vi "Write and Read Multiple Registers.vi"(4 "read count":u16, 6 "read starting address":u16, 8 "error in":errorcluster, 9 "write values":u16[](array[numeric]), 10 "write starting address":u16, 11 "device data model in":refnum<class "Standard Data Model.lvclass">) -> (0 "error out":errorcluster, 1 "read values":u16[](array[numeric]), 3 "device data model out":refnum<class "Standard Data Model.lvclass">)   [LabVIEW 2013, in "Modbus Library - Advance.lvlib" / "Standard Data Model.lvclass"]
doc: "Writes and reads the values of multiple register values in series. The <b>write values</b> are inserted starting at <b>write starting address</b> and the returned <b>read values</b> consists of <b>read count</b> holding registers starting at <b>read starting address</b>."
uses:
  Standard Data Model.lvclass
  Standard Data Model.lvclass/Standard Data Model.ctl
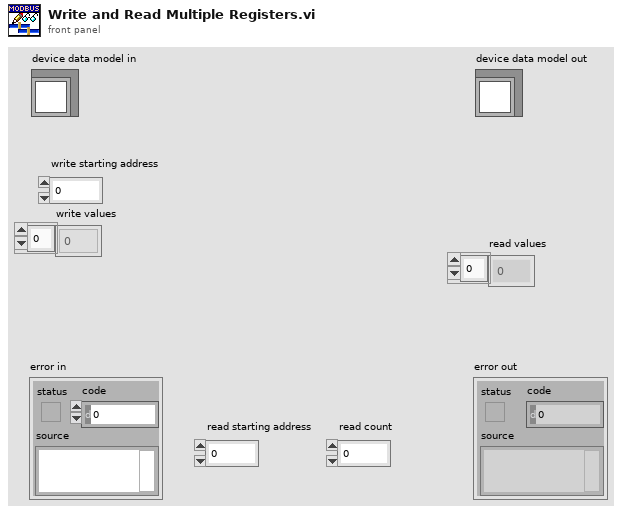
[diagram p1: front panel]
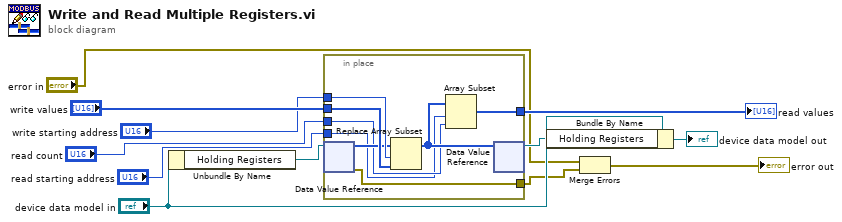
[diagram p0: block diagram]
diagram:
  n1 = Unbundle By Name("device data model in") -> ("Holding Registers"=w10:refnum<data-value>)
  n2 = in-place {
    in-place-border: "write values" -> [w20]
    in-place-border: "write starting address" -> [w19]
    in-place-border: [w16] -> w7
    in-place-border: "read count" -> [w15]
    in-place-border: "read starting address" -> [w14]
    in-place-border: [w13] -> w1
    n3 = in-place-dvr #1(w10) -> (w18:u16[], w13:errorcluster)
    n4 = Replace Array Subset(array=w18, new element=w20, index=w19) -> (w17:u16[])
    n5 = Array Subset(array=w17, index=w14, length=w15) -> (w16:u16[])
    n6 = in-place-dvr #1(w17) -> (w3:refnum<data-value>)  [unwired: 1 out]
  }
  "read values" <- w7
  n7 = Bundle By Name(cluster="device data model in", "Holding Registers"=w3) -> (→"device data model out":refnum<class "Standard Data Model.lvclass">)
  n8 = Merge Errors("error in", w1) -> (→"error out":errorcluster)
